vi "Read Applied Settings.vi"(8 "error in (no error)":errorcluster, 11 "UI Data in":refnum<class "Settings UI.lvclass">) -> (0 "error out":errorcluster, 2 "Applied Settings":T1={"Plug-in Version"="", "Step Values"=[], "Only Execute When Test Running"=TRUE, "Reset Sequence When Test Starts"=TRUE, "Number of Sequence Steps"=0, "Num of Analog Channels"=0, "Num of Digital Channels"=0, "Delay Before Starting Sequence"=0.0, "Default Analog Values"=[], "Default Digital Values"=[], "Max Iterations"=0, "Use last value when stopped"=FALSE, "Prioritize exact values"=FALSE, "Enable advanced step timing"=FALSE, "Enable step conditions"=FALSE, "Show confirmation dialogs"=FALSE, "Start condition"="", "Enable re-triggering"=FALSE, "Stop condition"=""}, 3 "UI Data out":refnum<class "Settings UI.lvclass">)   [LabVIEW 2020, in "Output Sequencer.lvlib" / "Settings UI.lvclass"]
uses:
  Settings UI.lvclass
  Types/Settings.ctl
  Types/Step Settings.ctl
  Settings UI.lvclass/Settings UI.ctl
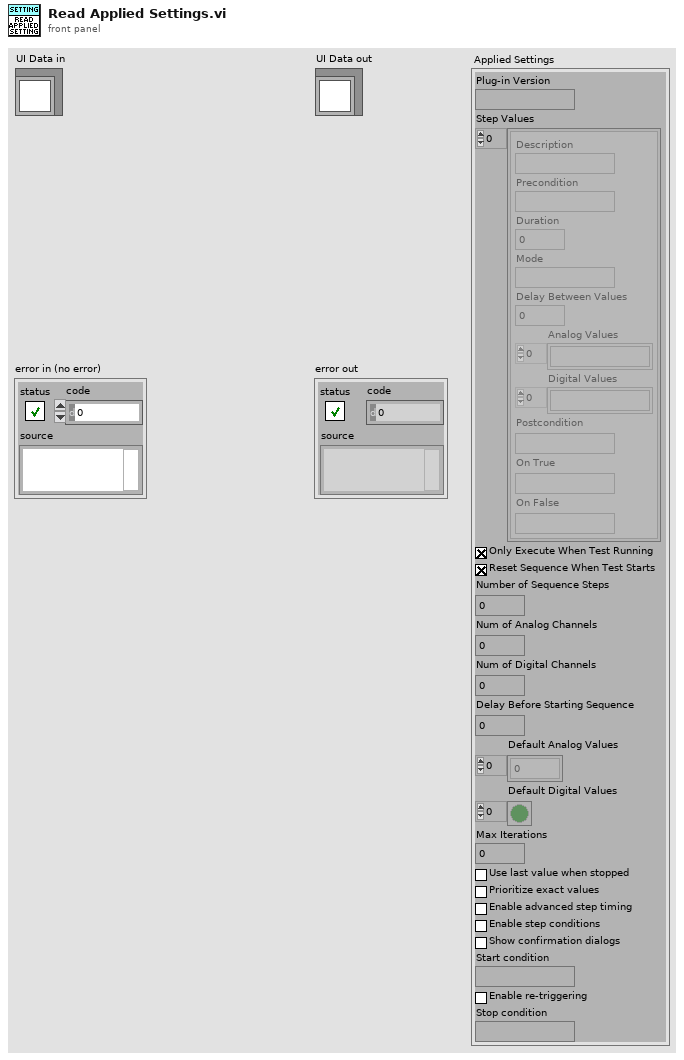
[diagram p1: front panel]
types:
  T1 = typedef "Output Sequencer.lvlib/Settings UI.lvclass/Settings.ctl" = cluster{"Plug-in Version":string, "Step Values":T2[], "Only Execute When Test Running":bool, "Reset Sequence When Test Starts":bool, "Number of Sequence Steps":i32, "Num of Analog Channels":i32, "Num of Digital Channels":i32, "Delay Before Starting Sequence":dbl, "Default Analog Values":dbl[], "Default Digital Values":bool[], "Max Iterations":u32, "Use last value when stopped":bool, "Prioritize exact values":bool, "Enable advanced step timing":bool, "Enable step conditions":bool, "Show confirmation dialogs":bool, "Start condition":string, "Enable re-triggering":bool, "Stop condition":string}
  T2 = typedef "Output Sequencer.lvlib/Settings UI.lvclass/Step Settings.ctl" = cluster{"Description":string, "Precondition":string, "Duration":dbl, "Mode":string, "Delay Between Values":dbl, "Analog Values":string[], "Digital Values":string[], "Postcondition":string, "On True":string, "On False":string}
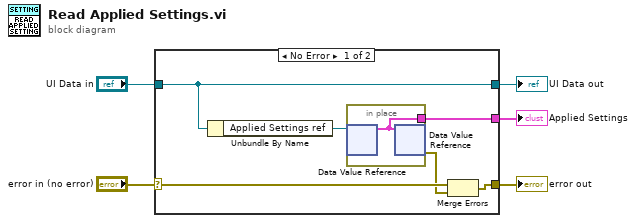
[diagram p0: block diagram]
diagram:
  n1 = case shown="No Error" "error in (no error)" {
    selector: "error in (no error)" -> [w8 w13]
    tunnel: [w6 w13] -> w4
    tunnel: [w11 w14] -> w2
    tunnel: "UI Data in" -> [w11 w14]
    tunnel: [w9 _] -> w1
    frame No Error {
      n2 = Unbundle By Name(w11) -> ("Applied Settings ref"=w10:refnum<data-value>)
      n3 = in-place {
        in-place-border: [w12] -> w9
        n4 = in-place-dvr #1(w10) -> (w12:T1)  [unwired: 1 out]
        n5 = in-place-dvr #1(w12) -> (w7:errorcluster)  [unwired: 1 out]
      }
      n6 = Merge Errors(w8, w7) -> (w6:errorcluster)
    }
    frame Error {
    }
  }
  "error out" <- w4
  "UI Data out" <- w2
  "Applied Settings" <- w1
